vi "Object.vi"(4 "Position":cluster{"X":sgl, "Y":sgl, "Z":sgl}, 8 "error in (no error)":errorcluster, 10 "Name":string) -> (0 "error out":errorcluster, 3 "3D Object out":refnum<class "3D Object.lvclass">)   [LabVIEW 2015, in "3D Object.lvclass"]
uses:
  3D Object.lvclass
  3D Object.lvclass/3D Object.ctl
  <vilib>/picture/3D Picture Control/Object/Create Object (name).vi
  <vilib>/picture/3D Picture Control/NI_3D Picture Control.lvlib
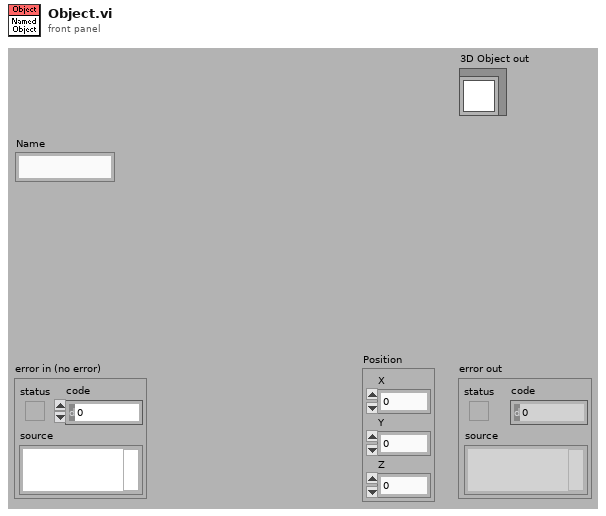
[diagram p1: front panel]
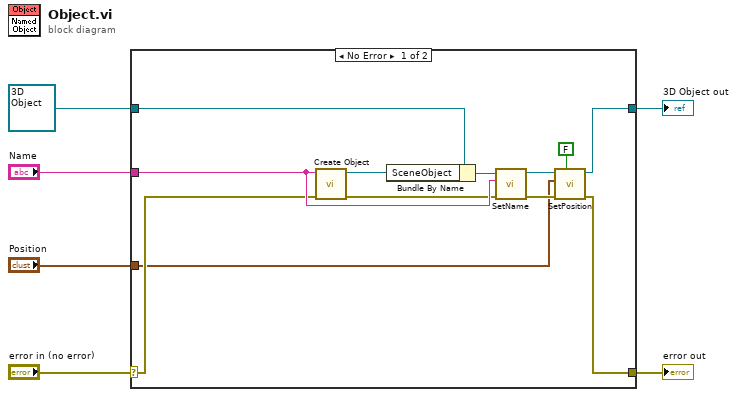
[diagram p0: block diagram]
diagram:
  n1 = case shown="No Error" "error in (no error)" {
    selector: "error in (no error)" -> [w10 w20]
    tunnel: [w17 w20] -> w5
    tunnel: [w7 w19] -> w3
    tunnel: refnum<class "3D Object.lvclass"> refnum ("3D Object in") -> [w16 w19]
    tunnel: "Name" -> [w13 _]
    tunnel: "Position" -> [w9 _]
    frame No Error {
      n2 = call-poly <vilib>:"Create Object.vi"("error in (no error)"=w10, "Name"=w13) -> ("error out"=w12:errorcluster, "Scene:New Object"=w18:refnum<vi>)  [unwired: 8 in]
      n3 = Bundle By Name(cluster=w16, "SceneObject"=w18) -> (w15:refnum<class "3D Object.lvclass">)
      n4 = call "SetName.vi"("error in (no error)"=w12, "Name"=w13, "3D Object in"=w15) -> ("error out"=w11:errorcluster, "3D Object out"=w14:refnum<class "3D Object.lvclass">)  [unwired: 7 out]
      n5 = call "SetPosition.vi"("Relative?"=FALSE, "error in (no error)"=w11, "Position"=w9, "3D Object in"=w14) -> ("error out"=w17:errorcluster, "3D Object out"=w7:refnum<class "3D Object.lvclass">)  [unwired: 6 in]
    }
    frame Error {
    }
  }
  "error out" <- w5
  "3D Object out" <- w3
